vi "pco.camera_FloatingMean_Example.vi"() -> ()   [LabVIEW 2019]
uses:
  pco.camera/Camera.lvclass
  <vilib>/picture/picture.llb/Draw True-Color Pixmap.vi
  <vilib>/picture/picture.llb/Draw 8-Bit Pixmap.vi
panel:
  out "colormap(U8)":u32[](array[numeric])
  in  "Zoom [%]":i32(c297)=26
  out "Image":picture
  out "Image(U16)":u16[][](graph)
  in  "averageCount":u8=10 caption="Average Count" min=2
  in  "data_format":T1(ring)=enum."Mono16"
  out "Recorded Images":u32
  in  "Quit":bool
  in  "roiY1":u64=2048 min=1 max=2160 step=1
  in  "roiX1":u64=2048 min=1 max=2560 step=1
  in  "roiY0":u64=1 min=1 max=2159 step=1
  in  "roiX0":u64=1 min=1 max=2559 step=1
  out "Image Height":u64
  out "Image Width":u64
  in  "dwImgCount":u32=10 caption="Fifo Buffer Size" max=4023
  out "Error":errorcluster {"code" format="%x"}
  # "This example shows how to compute and show a floating mean live image.\nHere the camera class is operated in fifo mode to always get next image in buffer.\nThe Average Count defines the number of images that will be averaged.\nAveraging is done by fetiching one image and using average image from previous iteration\n(avg_n = (1-1/avg_count)*avg_(n-1) + (1/avg_count)*image_n)\n\nIt is a good starting point for writing own applications.\nBut it will not be fail save, i.e. doesnt react on errors, just handles them forward to the end\n\nUsage:\nSelect your required fifo buffer size and image format and start the program.\nOnce started, the camera class will be initialized and image record will start automatically.\nInside the acquisition loop the program calculates the floating average image shows it.\nThe average count can be changed at any time.\nBy using the ROI parameters you can crop the image to select certain regions\n\nBy clicking Quit Application the record will stop and will force an exit of the camera class"
  # "pco.labview"
  # "Camera Setup"
  # "Recording Control"
  # "Parameters for image readout"
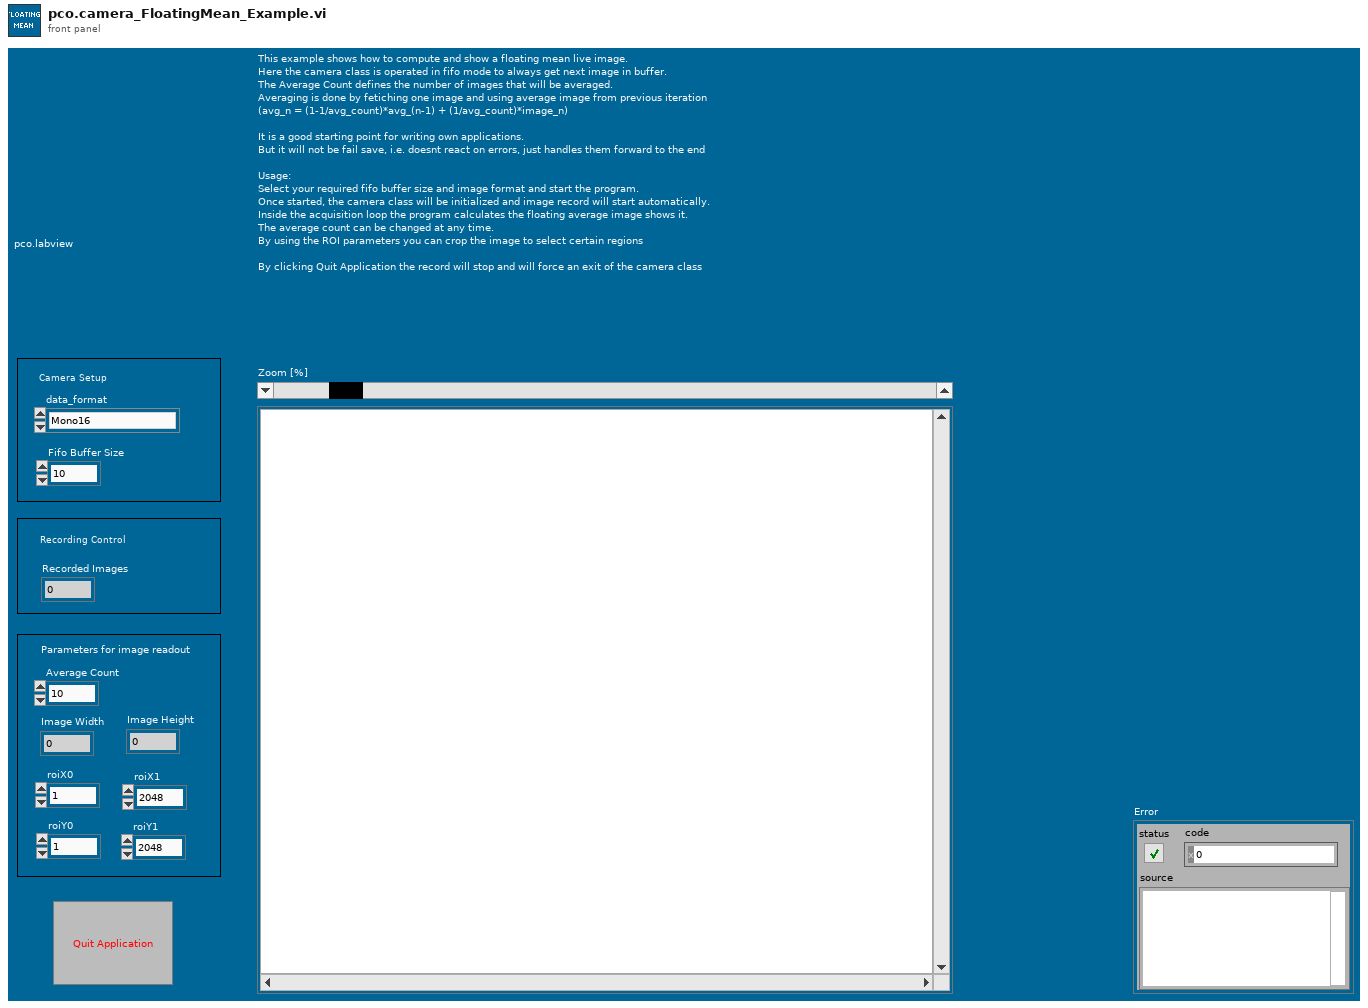
[diagram p1: front panel]
types:
  T1 = enum16{"Undefined", "Mono8", "Mono16", "BGRA8", "RGBA8", "BGRA16", "RGBA16", "CompressedMono8"}
  T2 = enum8{"Enabled", "Disabled", "Disabled and Grayed Out"}
  T3 = enum16{"sequence", "sequence non blocking", "ring buffer", "fifo", "sequence_dpcore", "sequence_non_blocking_dpcore", "ring_buffer_dpcore", "fifo_dpcore", "tif", "multitif", "pcoraw", "b16", "dicom", "multidicom"}
  T4 = typedef "Camera.lvclass/binning.ctl" = cluster{"vert":u16, "horz":u16}
  T5 = cluster{"exposure_time_s":dbl, "delay_time_s":dbl, "roi":cluster{"x0":u64, "y0":u64, "x1":u64, "y1":u64}, "timestamp_mode":u16, "pixelrate":u32, "trigger_mode":u16, "acquire_mode":u16, "metadata_mode":u16, "noisefilter_mode":u16, "binning":T4}
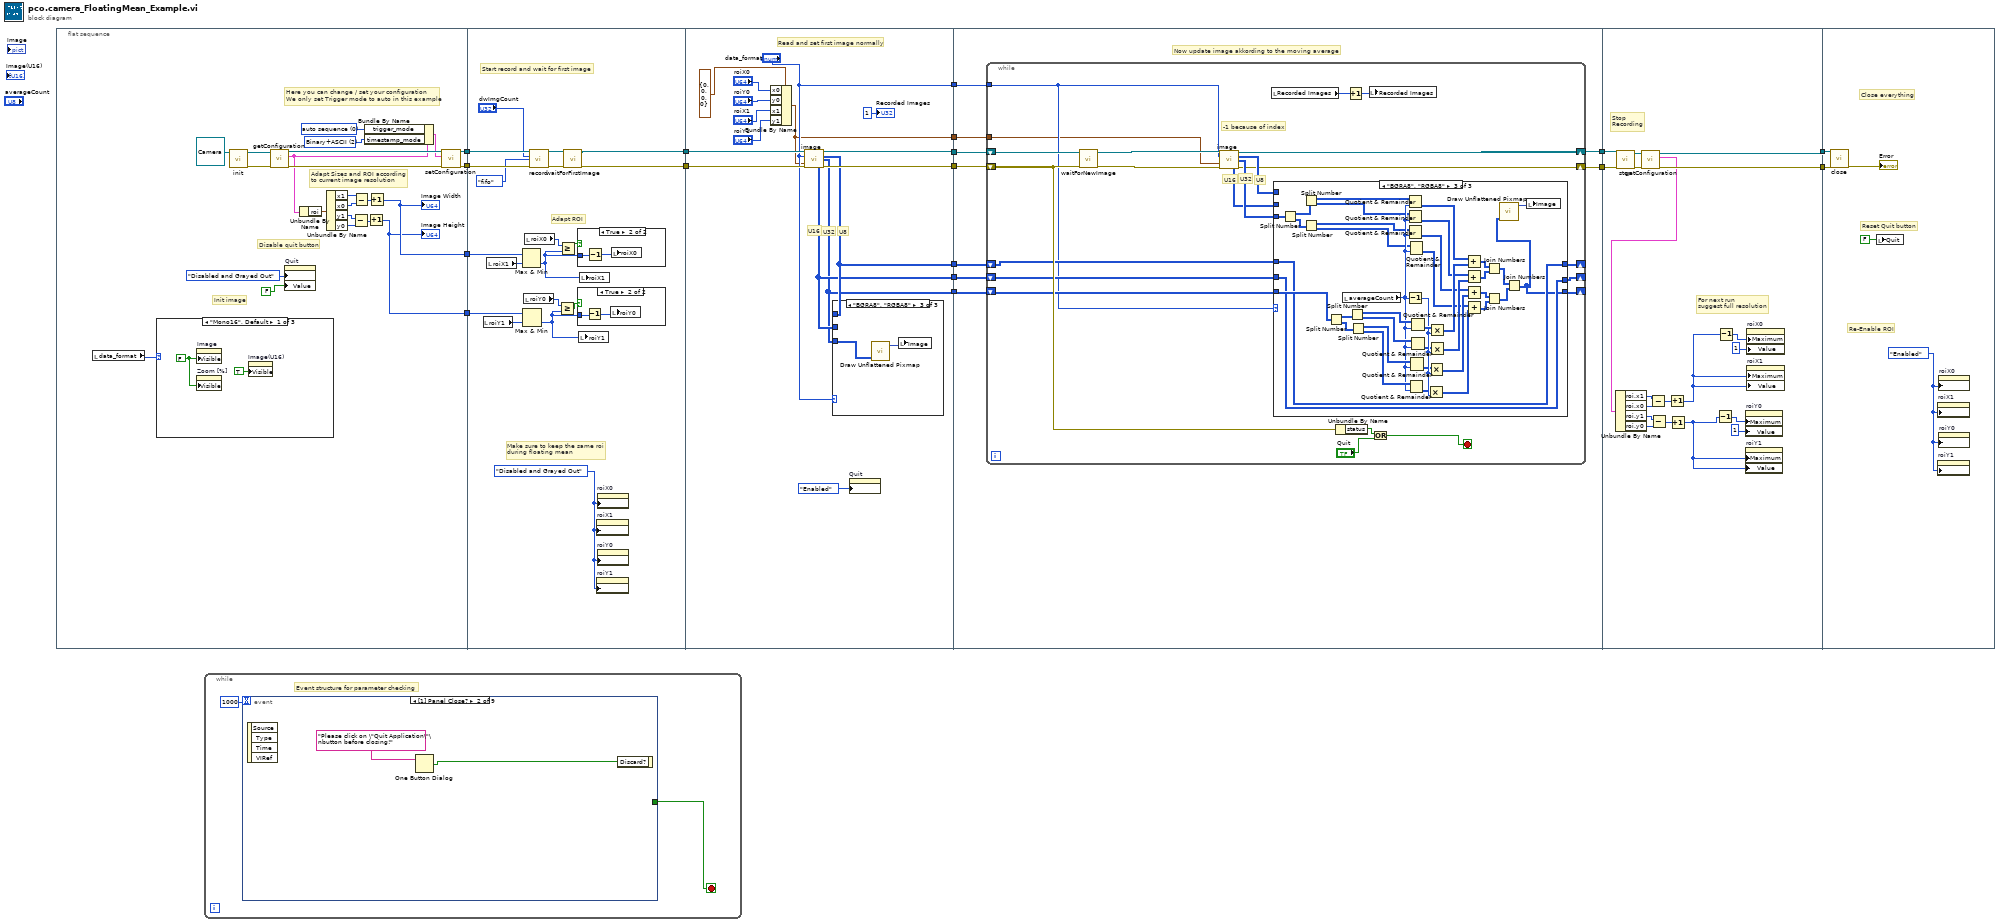
[diagram p0: block diagram]
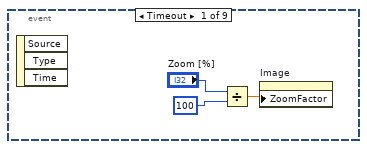
[diagram p2: hidden frame]
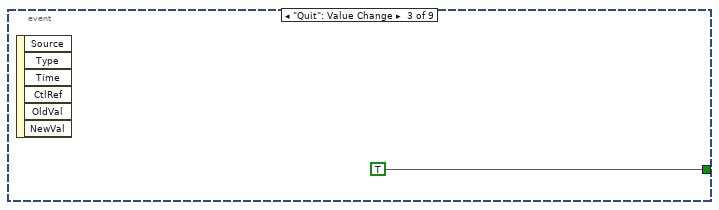
[diagram p3: hidden frame]
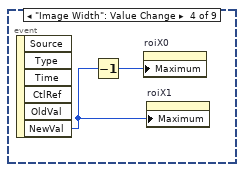
[diagram p4: hidden frame]
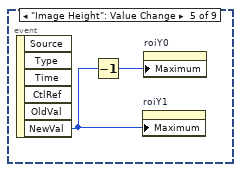
[diagram p5: hidden frame]
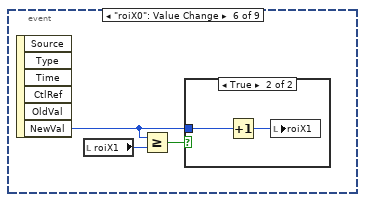
[diagram p6: hidden frame]
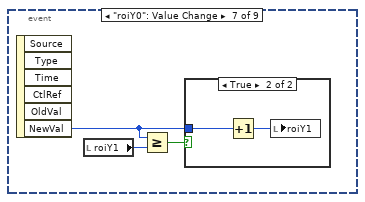
[diagram p8: hidden frame]
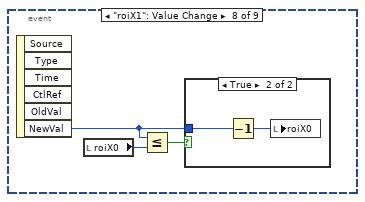
[diagram p10: hidden frame]
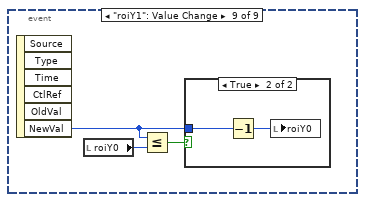
[diagram p12: hidden frame]
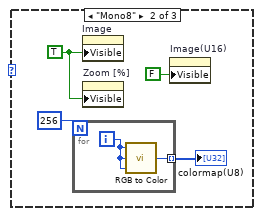
[diagram p14: hidden frame]
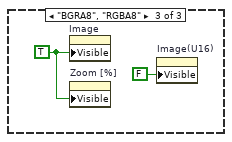
[diagram p15: hidden frame]
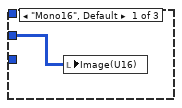
[diagram p18: hidden frame]
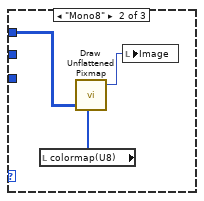
[diagram p19: hidden frame]
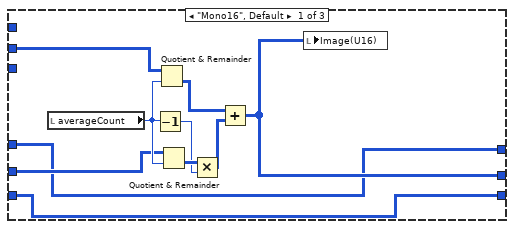
[diagram p20: hidden frame]
diagram:
  n1 = flat-sequence {
    tunnel: [w33] -> w17
    tunnel: [w32] -> w16
    tunnel: [w19] -> w2
    tunnel: [w18] -> w1
    tunnel: w17 -> [w69]
    tunnel: w16 -> [w68]
    tunnel: [w63] -> w15
    tunnel: [w62] -> w14
    tunnel: w2 -> [w52]
    tunnel: w1 -> [w51]
    tunnel: w15 -> [w88]
    tunnel: w14 -> [w87]
    tunnel: [w84] -> w13
    tunnel: [w85] -> w12
    tunnel: ["data_format"] -> w7
    tunnel: [w82] -> w6
    tunnel: [w81] -> w5
    tunnel: [w80] -> w4
    tunnel: [w74] -> w3
    tunnel: w13 -> [w103]
    tunnel: w12 -> [w104]
    tunnel: [w102] -> w11
    tunnel: [w101] -> w9
    tunnel: w7 -> [w100]
    tunnel: w6 -> [w99]
    tunnel: w5 -> [w98]
    tunnel: w4 -> [w97]
    tunnel: w3 -> [w96]
    tunnel: w11 -> [w205]
    tunnel: [w200] -> w10
    tunnel: w9 -> [w204]
    tunnel: [w201] -> w8
    tunnel: w10 -> [w208]
    tunnel: w8 -> [w207]
    frame #0 {
      w23 = u16 2 items=["OFF", "Binary", "Binary+ASCII", "ASCII"] ("TimestampMode")
      w37 = u16 0 items=["auto sequence"=0, "software trigger"=1, "external exposure start & software trigger"=2, "external exposure control"=3, "external synchronized"=4, "fast external exposure control"=5, "external CDS control"=6, "slow external exposure control"=7, "external synchronized HDSDI"=258] ("TriggerMode")
      # "Init image"
      # "Adapt Sizes and ROI according\nto current image resolution"
      # "Disable quit button"
      # "Here you can change / set your configuration\nWe only set Trigger mode to auto in this example"
      n2 = local read "data_format"() -> (w20:T1)
      n3 = case shown="\"Mono16\", Default" w20 {
        frame "Mono16", Default {
          w41 = FALSE ("Visible")
          n4 = property on="Image" class="Pict"("Visible"=w41) -> ()  [unwired: 2 in, 2 out]
          n5 = property on="Zoom [%]" class="Scroll (strict)"("Visible"=w41) -> ()  [unwired: 2 in, 2 out]
          n6 = property on="Image(U16)" class="IntGraph (strict)"("Visible"=TRUE) -> ()  [unwired: 2 in, 2 out]
        }
        frame "Mono8" {
          w45 = TRUE ("Visible")
          n7 = for {
            N: 256 -> [_]
            tunnel: [w47] -> w44 mode=indexing
            i -> [w48]
            n8 = call <vilib>:"RGB to Color.vi"("B"=w48, "G"=w48, "R"=w48) -> ("Color"=w47:u32)
          }
          "colormap(U8)" <- w44
          n9 = property on="Image" class="Pict"("Visible"=w45) -> ()  [unwired: 2 in, 2 out]
          n10 = property on="Zoom [%]" class="Scroll (strict)"("Visible"=w45) -> ()  [unwired: 2 in, 2 out]
          n11 = property on="Image(U16)" class="IntGraph (strict)"("Visible"=FALSE) -> ()  [unwired: 2 in, 2 out]
        }
        frame "BGRA8", "RGBA8" {
          w49 = TRUE ("Visible")
          n12 = property on="Image" class="Pict"("Visible"=w49) -> ()  [unwired: 2 in, 2 out]
          n13 = property on="Zoom [%]" class="Scroll (strict)"("Visible"=w49) -> ()  [unwired: 2 in, 2 out]
          n14 = property on="Image(U16)" class="IntGraph (strict)"("Visible"=FALSE) -> ()  [unwired: 2 in, 2 out]
        }
      }
      n15 = call-dynamic "init.vi"("Camera in"=refnum<class "Camera.lvclass"> refnum ("PCOCamera in")) -> ("Camera out"=w39:refnum<class "Camera.lvclass">, "error out"=w38:errorcluster)  [unwired: 8 in]
      n16 = call-dynamic "getConfiguration.vi"("error in (no error)"=w38, "Camera in"=w39) -> ("error out"=w35:errorcluster, "configuration"=w31:T5, "Camera out"=w36:refnum<class "Camera.lvclass">)  [unwired: 7 in]
      n17 = property on="Quit" class="Bool (strict)"("DisabledEnum"=T2."Disabled and Grayed Out" ("Disabled"), "Value"=FALSE ("Stop")) -> ()  [unwired: 2 in, 2 out]
      n18 = Unbundle By Name(w31) -> ("roi"=w30:cluster{"x0":u64, "y0":u64, "x1":u64, "y1":u64})
      n19 = Unbundle By Name(w30) -> ("x1"=w28:u64, "x0"=w29:u64, "y1"=w26:u64, "y0"=w27:u64)
      n20 = Subtract(x=w26, y=w27) -> (x-y=w24:u64)
      n21 = Subtract(x=w28, y=w29) -> (x-y=w25:u64)
      n22 = Bundle By Name(cluster=w31, "trigger_mode"=w37, "timestamp_mode"=w23) -> (w34:T5)
      n23 = Increment(x=w24) -> (x+1=w18:u64)
      "Image Height" <- w18
      n24 = Increment(x=w25) -> (x+1=w19:u64)
      "Image Width" <- w19
      n25 = call-dynamic "setConfiguration.vi"("error in (no error)"=w35, "configuration"=w34, "Camera in"=w36) -> ("error out"=w32:errorcluster, "Camera out"=w33:refnum<class "Camera.lvclass">)  [unwired: 7 in]
    }
    frame #1 {
      w61 = T2."Disabled and Grayed Out" ("Disabled")
      # "Adapt ROI"
      # "Make sure to keep the same roi\nduring floating mean"
      # "Start record and wait for first image"
      n26 = local read "roiY1"() -> (w59:u64)
      n27 = local read "roiX1"() -> (w60:u64)
      n28 = Max & Min(x=w52, y=w60) -> (min(x,y)=w56:u64)  [unwired: 1 out]
      n29 = Max & Min(x=w51, y=w59) -> (min(x,y)=w53:u64)  [unwired: 1 out]
      n30 = local read "roiY0"() -> (w54:u64)
      n31 = local read "roiX0"() -> (w58:u64)
      n32 = call-dynamic "record.vi"("Camera in"=w69, "num_images"="dwImgCount", "record_mode"=T3."fifo", "error in (no error)"=w68) -> ("Camera out"=w64:refnum<class "Camera.lvclass">, "error out"=w65:errorcluster)  [unwired: 10 in]
      n33 = Greater Or Equal?(x=w54, y=w53) -> (x >= y?=w55:bool)
      n34 = Greater Or Equal?(x=w58, y=w56) -> (x >= y?=w57:bool)
      n35 = call-dynamic "waitForFirstImage.vi"("error in (no error)"=w65, "Camera in"=w64) -> ("error out"=w62:errorcluster, "Camera out"=w63:refnum<class "Camera.lvclass">)  [unwired: 8 in]
      n36 = case shown="True" w55 {
        tunnel: w53 -> [_ w71]
        frame False {
        }
        frame True {
          n37 = Decrement(x=w71) -> (x-1=w70:u64)
          n38 = local write "roiY0"(w70) -> ()
        }
      }
      n39 = case shown="True" w57 {
        tunnel: w56 -> [_ w73]
        frame False {
        }
        frame True {
          n40 = Decrement(x=w73) -> (x-1=w72:u64)
          n41 = local write "roiX0"(w72) -> ()
        }
      }
      n42 = local write "roiY1"(w53) -> ()
      n43 = local write "roiX1"(w56) -> ()
      n44 = property on="roiX1" class="DigNum (strict)"("DisabledEnum"=w61) -> ()  [unwired: 2 in, 2 out]
      n45 = property on="roiY1" class="DigNum (strict)"("DisabledEnum"=w61) -> ()  [unwired: 2 in, 2 out]
      n46 = property on="roiX0" class="DigNum (strict)"("DisabledEnum"=w61) -> ()  [unwired: 2 in, 2 out]
      n47 = property on="roiY0" class="DigNum (strict)"("DisabledEnum"=w61) -> ()  [unwired: 2 in, 2 out]
    }
    frame #2 {
      # "U32"
      # "U8"
      # "U16"
      # "Read and set first image normally"
      n48 = Bundle By Name(cluster=cluster{"x0":u64, "y0":u64, "x1":u64, "y1":u64} {"x0"=0, "y0"=0, "x1"=0, "y1"=0} ("roi"), "x0"="roiX0", "y0"="roiY0", "x1"="roiX1", "y1"="roiY1") -> (w74:cluster{"x0":u64, "y0":u64, "x1":u64, "y1":u64})
      n49 = call-dynamic "image.vi"("Camera in"=w88, "data_format"="data_format", "roi"=w74, "error in (no error)"=w87) -> ("Camera out"=w84:refnum<class "Camera.lvclass">, "image (U8)"=w82:u8[][], "image (U32)"=w80:u32[][], "raw_image (U16)"=w81:u16[][], "error out"=w85:errorcluster)  [unwired: 4 in, 3 out]
      n50 = case shown="\"BGRA8\", \"RGBA8\"" "data_format" {
        tunnel: w80 -> [_ _ w95]
        tunnel: w82 -> [_ w93 _]
        tunnel: w81 -> [w90 _ _]
        frame "Mono16", Default {
          n51 = local write "Image(U16)"(w90) -> ()
        }
        frame "Mono8" {
          n52 = local read "colormap(U8)"() -> (w91:u32[])
          n53 = call-poly <vilib>:"Draw Unflattened Pixmap.vi"("data"=w93, "color table"=w91) -> ("new picture"=w92:picture)  [unwired: 7 in]
          n54 = local write "Image"(w92) -> ()
        }
        frame "BGRA8", "RGBA8" {
          n55 = call-poly <vilib>:"Draw Unflattened Pixmap.vi"("data (RGB format)"=w95) -> ("new picture"=w94:picture)  [unwired: 8 in]
          n56 = local write "Image"(w94) -> ()
        }
      }
      n57 = property on="Quit" class="Bool (strict)"("DisabledEnum"=T2."Enabled" ("Disabled")) -> ()  [unwired: 2 in, 2 out]
      "Recorded Images" <- u32 1 ("Recorded Images")
    }
    frame #3 {
      # "Now update image akkording to the moving average"
      n58 = while {
        shift-right: [w126] -> w102
        shift-left: w103 -> [w125]
        shift-right: [w106] -> w101
        shift-left: w104 -> [w120]
        tunnel: w100 -> [w109]
        shift-right: [w112] -> _
        shift-left: w99 -> [w116]
        shift-right: [w110] -> _
        shift-left: w98 -> [w115]
        shift-right: [w111] -> _
        shift-left: w97 -> [w114]
        tunnel: w96 -> [w105]
        stop <- w117 stop-if-true
        # "U8"
        # "-1 because of index"
        # "U32"
        # "U16"
        n59 = call-dynamic "waitForNewImage.vi"("error in (no error)"=w120, "Camera in"=w125) -> ("error out"=w121:errorcluster, "Camera out"=w122:refnum<class "Camera.lvclass">)  [unwired: 8 in]
        n60 = call-dynamic "image.vi"("Camera in"=w122, "data_format"=w109, "roi"=w105, "error in (no error)"=w121) -> ("Camera out"=w126:refnum<class "Camera.lvclass">, "image (U8)"=w113:u8[][], "image (U32)"=w108:u32[][], "raw_image (U16)"=w107:u16[][], "error out"=w106:errorcluster)  [unwired: 4 in, 3 out]
        n61 = local read "Recorded Images"() -> (w124:u32)
        n62 = case shown="\"BGRA8\", \"RGBA8\"" w109 {
          tunnel: w108 -> [_ _ w152]
          tunnel: w107 -> [w132 _ _]
          tunnel: w116 -> [w129 w146 w150]
          tunnel: w115 -> [w131 w138 w151]
          tunnel: w114 -> [w128 w137 w185]
          tunnel: w113 -> [_ w142 _]
          tunnel: [w129 w139 w150] -> w112
          tunnel: [w128 w137 w149] -> w111
          tunnel: [w130 w138 w151] -> w110
          frame "Mono16", Default {
            n63 = local read "averageCount"() -> (w135:u8)
            n64 = Decrement(x=w135) -> (x-1=w127:u8)
            n65 = Quotient & Remainder(x=w132, y=w135) -> (floor(x/y)=w134:u16[][])  [unwired: 1 out]
            n66 = Quotient & Remainder(x=w131, y=w135) -> (floor(x/y)=w136:u16[][])  [unwired: 1 out]
            n67 = Multiply(x=w136, y=w127) -> (x*y=w133:u16[][])
            n68 = Add(x=w134, y=w133) -> (x+y=w130:u16[][])
            n69 = local write "Image(U16)"(w130) -> ()
          }
          frame "Mono8" {
            n70 = local read "averageCount"() -> (w143:u8)
            n71 = Decrement(x=w143) -> (x-1=w144:u8)
            n72 = Quotient & Remainder(x=w142, y=w143) -> (floor(x/y)=w141:u8[][])  [unwired: 1 out]
            n73 = Quotient & Remainder(x=w146, y=w143) -> (floor(x/y)=w145:u8[][])  [unwired: 1 out]
            n74 = Multiply(x=w145, y=w144) -> (x*y=w140:u8[][])
            n75 = Add(x=w141, y=w140) -> (x+y=w139:u8[][])
            n76 = local read "colormap(U8)"() -> (w147:u32[])
            n77 = call-poly <vilib>:"Draw Unflattened Pixmap.vi"("data"=w139, "color table"=w147) -> ("new picture"=w148:picture)  [unwired: 7 in]
            n78 = local write "Image"(w148) -> ()
          }
          frame "BGRA8", "RGBA8" {
            n79 = Split Number(x=w152) -> (hi(x)=w173:u16[][], lo(x)=w172:u16[][])
            n80 = Split Number(x=w173) -> (hi(x)=w170:u8[][], lo(x)=w169:u8[][])
            n81 = Split Number(x=w172) -> (hi(x)=w168:u8[][], lo(x)=w167:u8[][])
            n82 = Split Number(x=w185) -> (hi(x)=w184:u16[][], lo(x)=w183:u16[][])
            n83 = local read "averageCount"() -> (w171:u8)
            n84 = Split Number(x=w184) -> (hi(x)=w181:u8[][], lo(x)=w176:u8[][])
            n85 = Split Number(x=w183) -> (hi(x)=w175:u8[][], lo(x)=w174:u8[][])
            n86 = Quotient & Remainder(x=w170, y=w171) -> (floor(x/y)=w166:u8[][])  [unwired: 1 out]
            n87 = Quotient & Remainder(x=w169, y=w171) -> (floor(x/y)=w164:u8[][])  [unwired: 1 out]
            n88 = Quotient & Remainder(x=w168, y=w171) -> (floor(x/y)=w160:u8[][])  [unwired: 1 out]
            n89 = Decrement(x=w171) -> (x-1=w180:u8)
            n90 = Quotient & Remainder(x=w167, y=w171) -> (floor(x/y)=w159:u8[][])  [unwired: 1 out]
            n91 = Quotient & Remainder(x=w174, y=w171) -> (floor(x/y)=w179:u8[][])  [unwired: 1 out]
            n92 = Quotient & Remainder(x=w175, y=w171) -> (floor(x/y)=w178:u8[][])  [unwired: 1 out]
            n93 = Quotient & Remainder(x=w181, y=w171) -> (floor(x/y)=w182:u8[][])  [unwired: 1 out]
            n94 = Quotient & Remainder(x=w176, y=w171) -> (floor(x/y)=w177:u8[][])  [unwired: 1 out]
            n95 = Multiply(x=w179, y=w180) -> (x*y=w161:u8[][])
            n96 = Multiply(x=w178, y=w180) -> (x*y=w162:u8[][])
            n97 = Multiply(x=w182, y=w180) -> (x*y=w165:u8[][])
            n98 = Multiply(x=w177, y=w180) -> (x*y=w163:u8[][])
            n99 = Add(x=w166, y=w165) -> (x+y=w158:u8[][])
            n100 = Add(x=w164, y=w163) -> (x+y=w157:u8[][])
            n101 = Add(x=w160, y=w162) -> (x+y=w156:u8[][])
            n102 = Add(x=w159, y=w161) -> (x+y=w155:u8[][])
            n103 = Join Numbers(hi=w158, lo=w157) -> ((hi.lo)=w154:u16[][])
            n104 = Join Numbers(hi=w156, lo=w155) -> ((hi.lo)=w153:u16[][])
            n105 = Join Numbers(hi=w154, lo=w153) -> ((hi.lo)=w149:u32[][])
            n106 = call-poly <vilib>:"Draw Unflattened Pixmap.vi"("data (RGB format)"=w149) -> ("new picture"=w186:picture)  [unwired: 8 in]
            n107 = local write "Image"(w186) -> ()
          }
        }
        n108 = Unbundle By Name(w120) -> ("status"=w119:bool)
        n109 = Increment(x=w124) -> (x+1=w123:u32)
        n110 = local write "Recorded Images"(w123) -> ()
        n111 = Or(x=w119, y="Quit") -> (x .or. y?=w117:bool)
      }
    }
    frame #4 {
      # "For next run \nsuggest full resolution"
      # "Stop \nRecording"
      n112 = call-dynamic "stop.vi"("error in (no error)"=w204, "Camera in"=w205) -> ("error out"=w202:errorcluster, "Camera out"=w203:refnum<class "Camera.lvclass">)  [unwired: 8 in]
      n113 = call-dynamic "getConfiguration.vi"("error in (no error)"=w202, "Camera in"=w203) -> ("error out"=w201:errorcluster, "configuration"=w199:T5, "Camera out"=w200:refnum<class "Camera.lvclass">)  [unwired: 7 in]
      n114 = Unbundle By Name(w199) -> ("roi.x1"=w193:u64, "roi.x0"=w194:u64, "roi.y1"=w195:u64, "roi.y0"=w196:u64)
      n115 = Subtract(x=w193, y=w194) -> (x-y=w192:u64)
      n116 = Subtract(x=w195, y=w196) -> (x-y=w191:u64)
      n117 = Increment(x=w192) -> (x+1=w188:u64)
      n118 = Increment(x=w191) -> (x+1=w189:u64)
      n119 = Decrement(x=w189) -> (x-1=w190:u64)
      n120 = Decrement(x=w188) -> (x-1=w187:u64)
      n121 = property on="roiY0" class="DigNum (strict)"("Maximum"=w190, "Value"=u64 1 ("roiY0")) -> ()  [unwired: 2 in, 2 out]
      n122 = property on="roiY1" class="DigNum (strict)"("Maximum"=w189, "Value"=w189) -> ()  [unwired: 2 in, 2 out]
      n123 = property on="roiX0" class="DigNum (strict)"("Maximum"=w187, "Value"=u64 1 ("roiX0")) -> ()  [unwired: 2 in, 2 out]
      n124 = property on="roiX1" class="DigNum (strict)"("Maximum"=w188, "Value"=w188) -> ()  [unwired: 2 in, 2 out]
    }
    frame #5 {
      w206 = T2."Enabled" ("Disabled")
      # "Re-Enable ROI"
      # "Reset Quit button"
      # "Close everything"
      n125 = call-dynamic "close.vi"("error in (no error)"=w207, "Camera in"=w208) -> ("error out"=→"Error":errorcluster)  [unwired: 9 in]
      n126 = local write "Quit"(FALSE ("Stop")) -> ()
      n127 = property on="roiX1" class="DigNum (strict)"("DisabledEnum"=w206) -> ()  [unwired: 2 in, 2 out]
      n128 = property on="roiY1" class="DigNum (strict)"("DisabledEnum"=w206) -> ()  [unwired: 2 in, 2 out]
      n129 = property on="roiX0" class="DigNum (strict)"("DisabledEnum"=w206) -> ()  [unwired: 2 in, 2 out]
      n130 = property on="roiY0" class="DigNum (strict)"("DisabledEnum"=w206) -> ()  [unwired: 2 in, 2 out]
    }
  }
  n131 = while {
    stop <- w211 stop-if-true
    # "Event structure for parameter checking"
    n132 = event shown="[1] Panel Close?" {
      selector: _ -> [_ _ _ _ _ _ _ _ _]
      dyn-events: _ -> [_ _ _ _ _ _ _ _ _]
      timeout: 1000 -> [_ _ _ _ _ _ _ _ _]
      tunnel: [_ _ TRUE _ _ _ _ _ _] -> w211
      event Timeout {
        n133 = event-data() -> ()  [unwired: 1 in, 3 out]
        n134 = Divide(x="Zoom [%]", y=100 ("Zoom [%]")) -> (x/y=w215:dbl)
        n135 = property on="Image" class="Pict"("ZoomFactor"=w215) -> ()  [unwired: 2 in, 2 out]
      }
      event Panel Close? {
        n136 = event-data() -> ()  [unwired: 1 in, 4 out]
        n137 = One Button Dialog(message="Please click on \"Quit Application\"\nbutton before closing!") -> (true=w216:bool)  [unwired: 1 in]
        n138 = event-data("Discard?"=w216) -> ()  [unwired: 1 in, 1 out]
      }
      event "Quit": Value Change {
        n139 = event-data() -> ()  [unwired: 1 in, 6 out]
      }
      event "Image Width": Value Change {
        n140 = event-data() -> ("NewVal"=w219:u64)  [unwired: 1 in, 5 out]
        n141 = Decrement(x=w219) -> (x-1=w220:u64)
        n142 = property on="roiX0" class="DigNum (strict)"("Maximum"=w220) -> ()  [unwired: 2 in, 2 out]
        n143 = property on="roiX1" class="DigNum (strict)"("Maximum"=w219) -> ()  [unwired: 2 in, 2 out]
      }
      event "Image Height": Value Change {
        n144 = event-data() -> ("NewVal"=w221:u64)  [unwired: 1 in, 5 out]
        n145 = Decrement(x=w221) -> (x-1=w222:u64)
        n146 = property on="roiY1" class="DigNum (strict)"("Maximum"=w221) -> ()  [unwired: 2 in, 2 out]
        n147 = property on="roiY0" class="DigNum (strict)"("Maximum"=w222) -> ()  [unwired: 2 in, 2 out]
      }
      event "roiX0": Value Change {
        n148 = event-data() -> ("NewVal"=w223:u64)  [unwired: 1 in, 5 out]
        n149 = local read "roiX1"() -> (w225:u64)
        n150 = Greater Or Equal?(x=w223, y=w225) -> (x >= y?=w224:bool)
        n151 = case shown="True" w224 {
          tunnel: w223 -> [_ w227]
          frame False {
          }
          frame True {
            n152 = Increment(x=w227) -> (x+1=w226:u64)
            n153 = local write "roiX1"(w226) -> ()
          }
        }
      }
      event "roiY0": Value Change {
        n154 = event-data() -> ("NewVal"=w228:u64)  [unwired: 1 in, 5 out]
        n155 = local read "roiY1"() -> (w230:u64)
        n156 = Greater Or Equal?(x=w228, y=w230) -> (x >= y?=w229:bool)
        n157 = case shown="True" w229 {
          tunnel: w228 -> [_ w232]
          frame False {
          }
          frame True {
            n158 = Increment(x=w232) -> (x+1=w231:u64)
            n159 = local write "roiY1"(w231) -> ()
          }
        }
      }
      event "roiX1": Value Change {
        n160 = event-data() -> ("NewVal"=w233:u64)  [unwired: 1 in, 5 out]
        n161 = local read "roiX0"() -> (w235:u64)
        n162 = Less Or Equal?(x=w233, y=w235) -> (x <= y?=w234:bool)
        n163 = case shown="True" w234 {
          tunnel: w233 -> [_ w237]
          frame False {
          }
          frame True {
            n164 = Decrement(x=w237) -> (x-1=w236:u64)
            n165 = local write "roiX0"(w236) -> ()
          }
        }
      }
      event "roiY1": Value Change {
        n166 = event-data() -> ("NewVal"=w238:u64)  [unwired: 1 in, 5 out]
        n167 = local read "roiY0"() -> (w240:u64)
        n168 = Less Or Equal?(x=w238, y=w240) -> (x <= y?=w239:bool)
        n169 = case shown="True" w239 {
          tunnel: w238 -> [_ w242]
          frame False {
          }
          frame True {
            n170 = Decrement(x=w242) -> (x-1=w241:u64)
            n171 = local write "roiY0"(w241) -> ()
          }
        }
      }
    }
  }
